vi "mode_generation_(subvi).vi"(0 "beam waist w0 (m) in":dbl=0.0001 format="%.2p", 2 "beam parameters in":T1, 3 "phase":dbl[](array[numeric]), 4 "coeffs":dbl[](array[numeric]), 5 "p":dbl[](array[numeric]) format="%#_13g", 6 "l":dbl[](array[numeric])) -> (1 "mode encoding":T1)   [LabVIEW 2015]
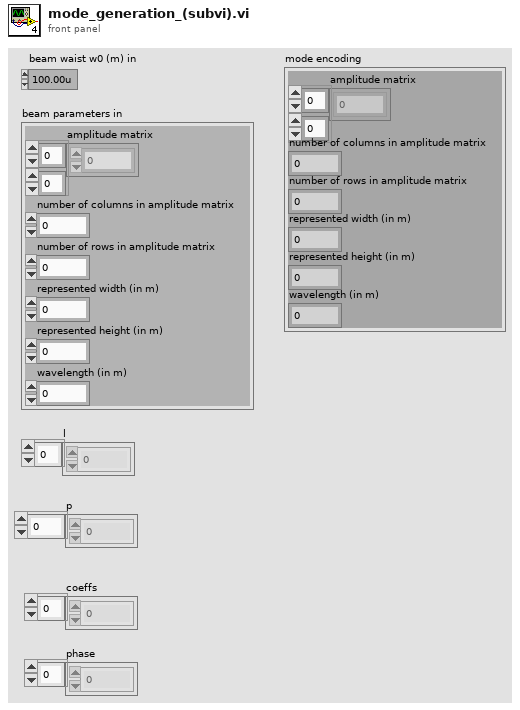
[diagram p1: front panel]
types:
  T1 = cluster{"amplitude matrix":cdb[][], "number of columns in amplitude matrix":i32, "number of rows in amplitude matrix":i32, "represented width (in m)":dbl, "represented height (in m)":dbl, "wavelength (in m)":dbl}
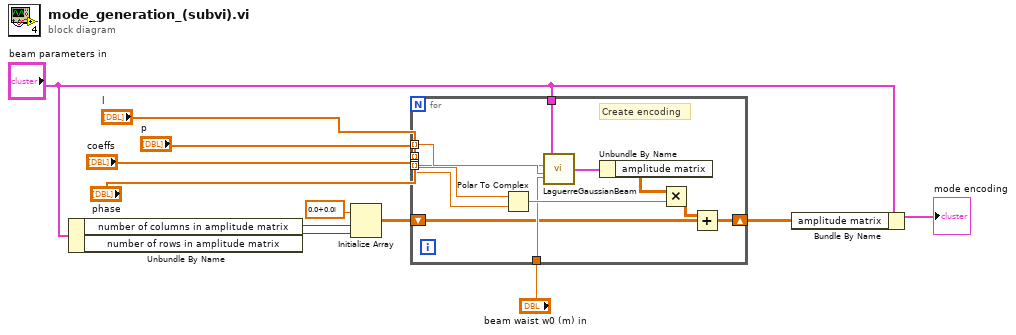
[diagram p0: block diagram]
diagram:
  n1 = Unbundle By Name("beam parameters in") -> ("number of columns in amplitude matrix"=w6:i32, "number of rows in amplitude matrix"=w5:i32)
  n2 = Initialize Array(cdb 0.0+0.0i ("element"), w6, w5) -> (w10:cdb[][])
  n3 = for {
    tunnel: "beam parameters in" -> [w22]
    tunnel: "beam waist w0 (m) in" -> [w21]
    shift-right: [w18] -> w9
    shift-left: w10 -> [w19]
    tunnel: "coeffs" -> [w15] mode=indexing
    tunnel: "phase" -> [w16] mode=indexing
    tunnel: "p" -> [w14] mode=indexing
    tunnel: "l" -> [w13] mode=indexing
    # "Create encoding"
    n4 = Polar To Complex(1:w16, 2:w15) -> (0:w23:cdb)
    n5 = call <userlib>:"LaguerreGaussianBeam.vi"("beam waist w0 (in m; default 1E-4 = 0.1mm)"=w21, "p"=w14, "l"=w13, "beam parameters"=w22) -> ("Laguerre-Gaussian beam"=w17:T1)  [unwired: 7 in]
    n6 = Unbundle By Name(w17) -> ("amplitude matrix"=w24:cdb[][])
    n7 = Multiply(x=w24, y=w23) -> (x*y=w20:cdb[][])
    n8 = Add(x=w20, y=w19) -> (x+y=w18:cdb[][])
  }
  n9 = Bundle By Name(cluster="beam parameters in", "amplitude matrix"=w9) -> (→"mode encoding":T1)
